vi "defineFinalRobotOrientaion.vi"(8 "error in (no error)":errorcluster, 10 "Robot":refnum<class "Robot.lvclass">, 11 "Game in":refnum<class "Game.lvclass">) -> (0 "error out":errorcluster, 2 "dest_orientation":dbl, 3 "Game out":refnum<class "Game.lvclass">)   [LabVIEW 2023, in "Game.lvclass"]
uses:
  Game.lvclass
  Robot_class/Robot.lvclass
  Robot_class/Robot.lvclass/Robot.ctl
  Robot_class/Read robotKickState.vi
  Robot_class/Read orientation.vi
  Robot_class/Read dest_orientation.vi
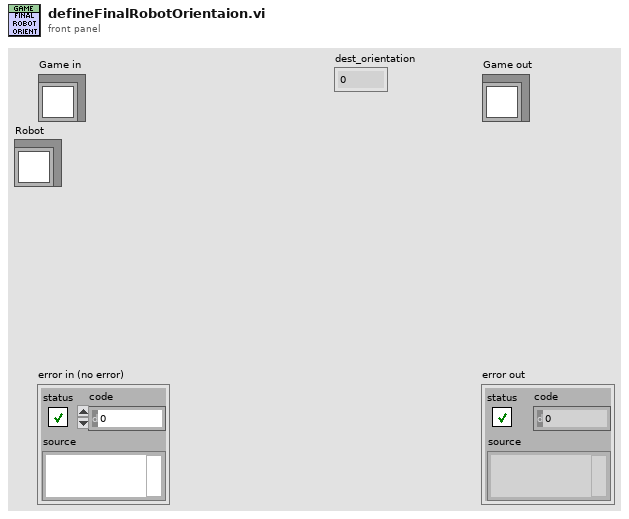
[diagram p1: front panel]
types:
  T1 = typedef "robotKickToStates.ctl" = enum16{"shootFromDirect", "avoidCollideBall", "goToBackBall", "none", "walk", "turn", "turnAntiClockWise", "turnClockwise", "oldKickToShoot", "oldKickToGoToBackBall", "shoot"}
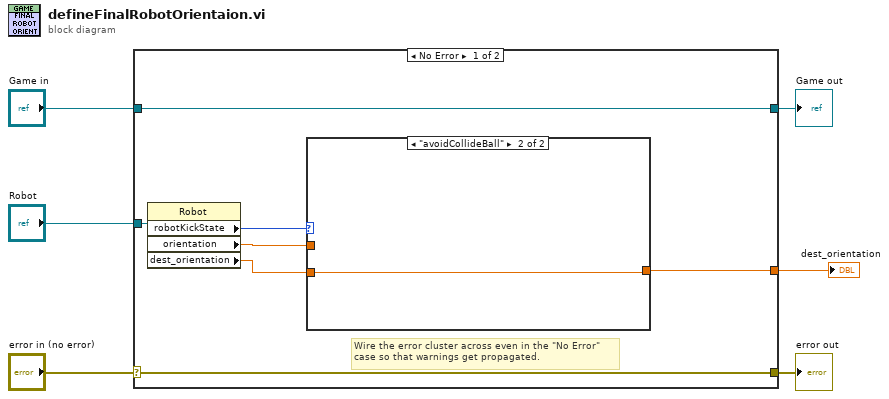
[diagram p0: block diagram]
diagram:
  n1 = case shown="No Error" "error in (no error)" {
    selector: "error in (no error)" -> [w12 w17]
    tunnel: [w12 w17] -> w5
    tunnel: [w13 w16] -> w3
    tunnel: "Game in" -> [w13 w16]
    tunnel: "Robot" -> [w11 _]
    tunnel: [w9 _] -> w1
    frame No Error {
      # "Wire the error cluster across even in the \"No Error\"\ncase so that warnings get propagated."
      n2 = property class="Robot"(reference=w11) -> ("robotKickState"=w8:T1, "orientation"=w7:dbl, "dest_orientation"=w10:dbl)  [unwired: 1 in, 2 out]
      n3 = case shown="\"avoidCollideBall\"" w8 {
        tunnel: [w14 w15] -> w9
        tunnel: w10 -> [w14 w15]
        tunnel: w7 -> [_ _]
        frame "none", Default {
          # "\"none\" para os robôs que não estão\nexecutando a kickTo.\nE default para os states \"girar\" e \"chutar\"\nda newKickTo"
        }
        frame "avoidCollideBall" {
        }
      }
    }
    frame Error {
    }
  }
  "error out" <- w5
  "Game out" <- w3
  "dest_orientation" <- w1
